vi "DMM_Verify Instrument Options - Versions.vi"(8 "error in (no error)":errorcluster, 11 "DMM Virtual in":refnum<class "DMM Virtual.lvclass">) -> (0 "error out":errorcluster, 3 "DMM Virtual out":refnum<class "DMM Virtual.lvclass">)   [LabVIEW 2018, in "DMM Virtual.lvclass"]
uses:
  DMM Virtual.lvclass
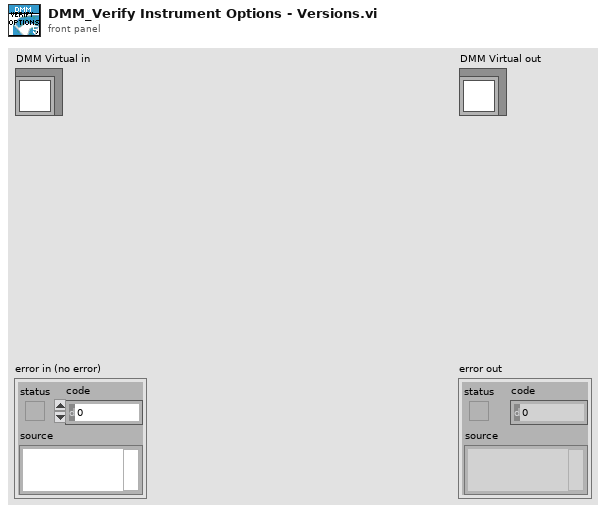
[diagram p1: front panel]
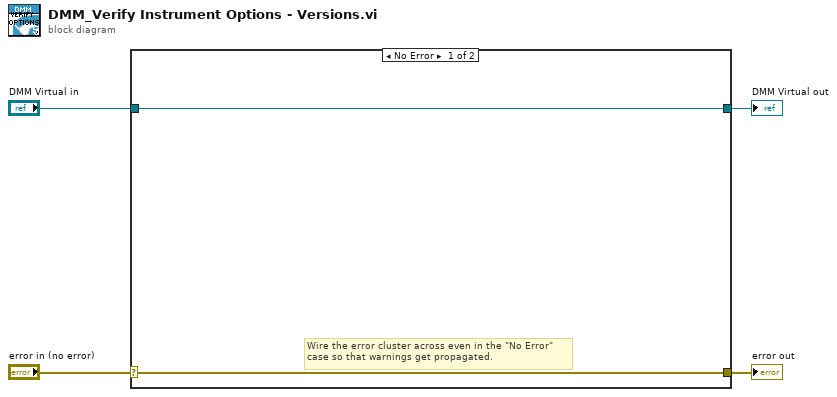
[diagram p0: block diagram]
diagram:
  n1 = case shown="No Error" "error in (no error)" {
    selector: "error in (no error)" -> [w5 w8]
    tunnel: [w5 w8] -> w3
    tunnel: [w6 w7] -> w1
    tunnel: "DMM Virtual in" -> [w6 w7]
    frame No Error {
      # "Wire the error cluster across even in the \"No Error\"\ncase so that warnings get propagated."
    }
    frame Error {
    }
  }
  "error out" <- w3
  "DMM Virtual out" <- w1
